vi "Disconnected.vi"(8 "error in (no error)":errorcluster, 10 "InstrumentData 2":T1, 11 "Camera_Controller in":refnum<class "Camera_Controller.lvclass">) -> (0 "error out":errorcluster, 3 "Camera_Controller out":refnum<class "Camera_Controller.lvclass">)   [LabVIEW 2023, in "Camera_Controller.lvlib" / "Camera_Controller.lvclass"]
uses:
  Camera_Controller.lvclass
  typedefs/InstrumentData.ctl
  <vilib>/ActorFramework/Message Enqueuer/Message Enqueuer.lvclass
  typedefs/instrumentType.ctl
  typedefs/typedefs.lvlib
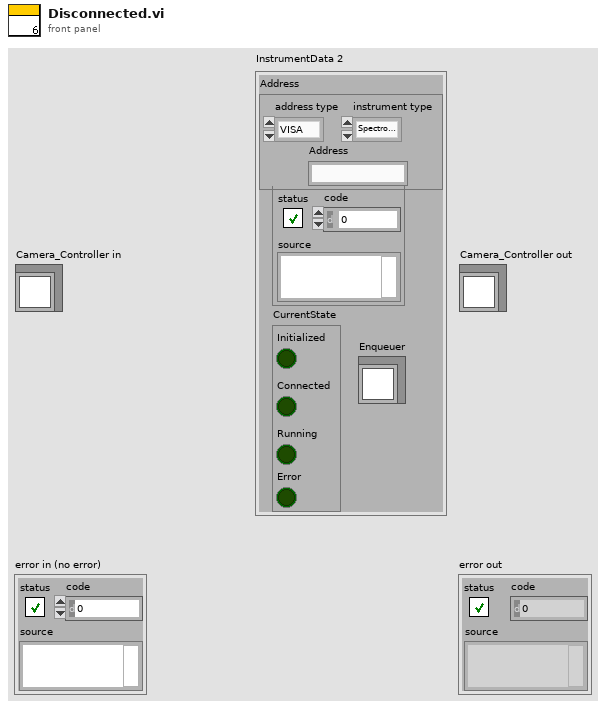
[diagram p1: front panel]
types:
  T1 = typedef "typedefs.lvlib/InstrumentData.ctl" = cluster{"Instr Error":errorcluster, "Address":cluster{"address type":enum16{"VISA", "Index"}, "Address":string, "instrument type":T2}, "CurrentState":cluster{"Initialized":bool, "Connected":bool, "Running":bool, "Error":bool}, "Enqueuer":refnum<class "Message Enqueuer.lvclass">}
  T2 = typedef "typedefs.lvlib/instrumentType.ctl" = enum16{"Spectrometer", "Camera", "Stepper", "Piezo"}
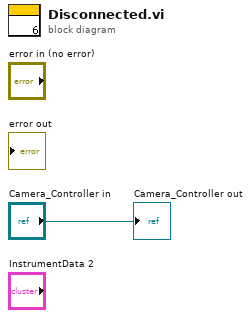
[diagram p0: block diagram]
diagram:
  "Camera_Controller out" <- "Camera_Controller in"
